vi "Memory.Size to Count.Power of 2.vi"(7 "power of 2":i16, 11 "size":u64 format="%08x bytes") -> (3 "count":u64 format="%0d")   [LabVIEW 2016, in "Memory Manager.lvlib"]
doc: "Downshifts <b>size</b> by the specified <b>power of 2</b> to get the count."
uses:
  Memory Manager.lvlib
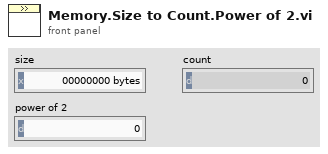
[diagram p1: front panel]
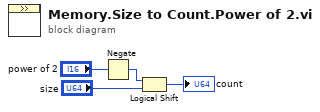
[diagram p0: block diagram]
diagram:
  n1 = Negate(x="power of 2") -> (-x=w1:i16)
  n2 = Logical Shift(y=w1, x="size") -> (x << y=→"count":u64)
